vi "Thermopower-v2.vi"(0 "Gate Start":dbl format="%#_13g", 1 "hold time (sec)":dbl=10.0 format="%#_13g", 2 "Gate step - extra milliseconds to wait":u32=20000, 4 "N Gate Intervals":i32=7, 5 "Gate Step":dbl=-6.0, 6 "N Heater Intervals":i32=7, 7 "Heater Step":dbl=3.3) -> ()   [LabVIEW 2016]
uses:
  <vilib>/Utility/file.llb/Write To Spreadsheet File (DBL).vi
  <vilib>/Utility/file.llb/Read From Spreadsheet File (DBL).vi
  Driver/New driver/Agilent 415X Series.lvlib
panel:
  out "Voltage across heater (VSU 1 and SMU4) 2":dbl[][](graph)
  out "error out 2":errorcluster
  out "Gate Voltage (SMU 3) 2":dbl[](graph)
  out "Thermal Voltage (SMU2), SMU1 is Common 2":dbl[](graph)
  out "SPA VISA resource name 2":refnum<visa-resource-name>
  out "Voltage across heater (VSU 1 and SMU4)":dbl[][](graph)
  out "Gate Voltage (SMU 3)":dbl[](graph)
  out "Thermal Voltage (SMU2), SMU1 is Common":dbl[](graph)
  in  "SPA VISA resource name":refnum<visa-resource-name>="GPIB0::14::INSTR"
  in  "error in (no error)":errorcluster
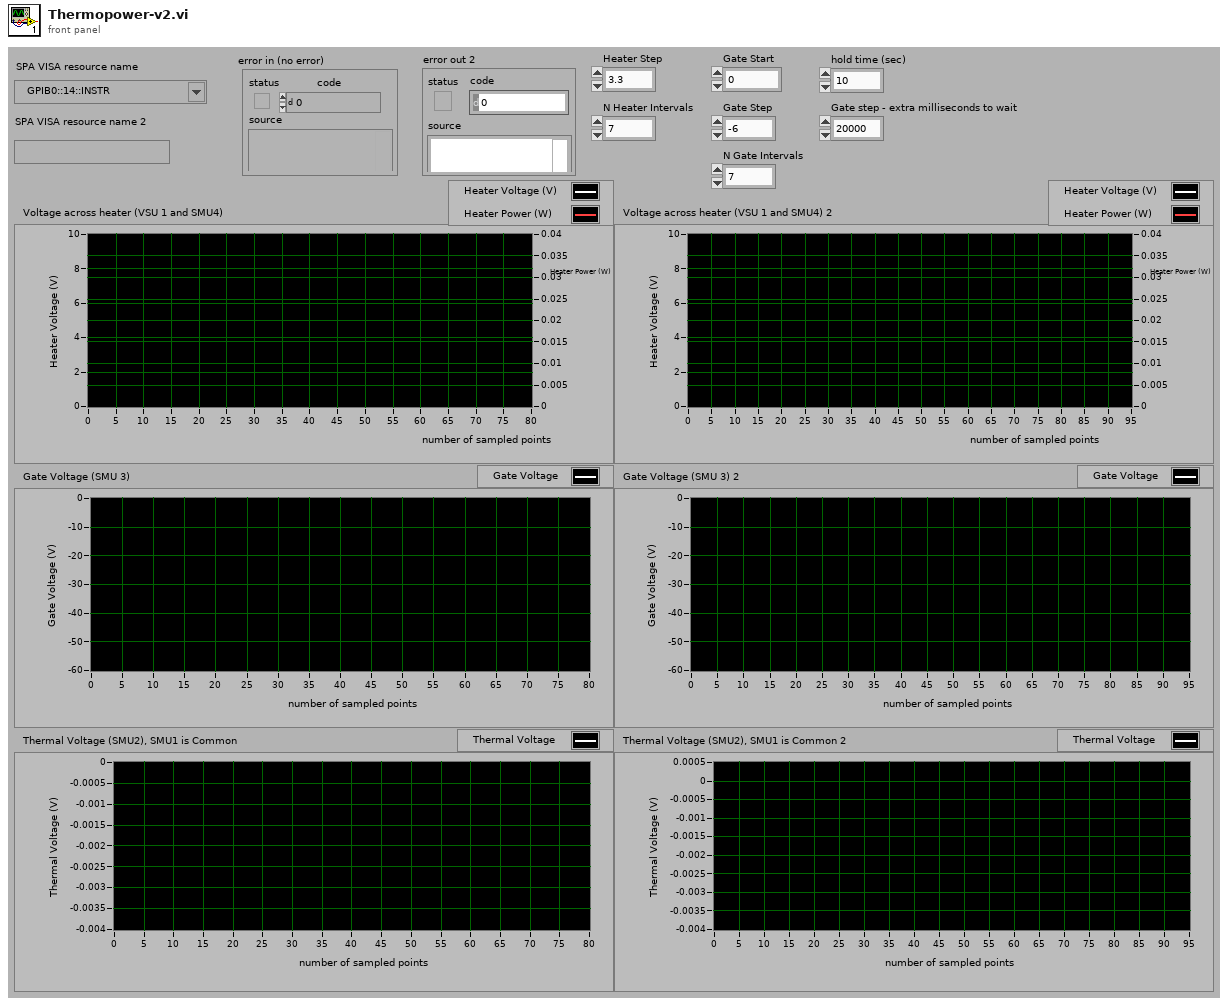
[diagram p1: front panel]
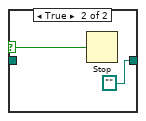
[diagram p3: hidden frame]
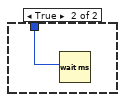
[diagram p4: hidden frame]
diagram:
  # "calculate end gate voltage"
  n1 = flat-sequence {
    tunnel: "error in (no error)" -> [w51]
    tunnel: "SPA VISA resource name" -> [w50]
    tunnel: [w49] -> w45
    tunnel: [w48] -> w44
    tunnel: w45 -> [w58]
    tunnel: w44 -> [w57]
    tunnel: [w54] -> w43
    tunnel: [w53] -> w42
    tunnel: w43 -> [w66]
    tunnel: w42 -> [w65]
    tunnel: [w64] -> w41
    tunnel: [w63] -> w40
    tunnel: w41 -> [w77]
    tunnel: w40 -> [w76]
    tunnel: [w75] -> w39
    tunnel: [w74] -> w38
    tunnel: w39 -> [w88]
    tunnel: w38 -> [w87]
    tunnel: [w86] -> w37
    tunnel: [w85] -> w35
    tunnel: w37 -> [w93]
    tunnel: [w94] -> w36
    tunnel: w35 -> [w92]
    tunnel: [w95] -> w34
    tunnel: w36 -> [w110]
    tunnel: w34 -> [w112]
    tunnel: [w111] -> w27
    tunnel: [w109] -> w26
    tunnel: w27 -> [w130]
    tunnel: w26 -> [w131]
    tunnel: [w115] -> w2
    tunnel: [w114] -> w1
    tunnel: [w133] -> w33
    tunnel: [w136] -> w32
    tunnel: [w135] -> w5
    tunnel: w2 -> [w133]
    tunnel: w1 -> [w134]
    frame #0 {
      n2 = call "Initialize.vi"("error in (no error)"=w51, "reset"=TRUE, "VISA resource name"=w50) -> ("error out"=w48:errorcluster, "VISA resource name out"=w49:refnum<visa-resource-name>)  [unwired: 2 in, 5 out]
    }
    frame #1 {
      n3 = call "Select-Meas. Mode.vi"("clear all channels"=TRUE, "error in (no error)"=w57, "measurement mode"=TRUE, "VISA resource name"=w58) -> ("error out"=w53:errorcluster, "VISA resource name out"=w54:refnum<visa-resource-name>)  [unwired: 1 in, 5 out]
    }
    frame #2 {
      w61 = 0 items=["0  ", "10K Ohms  ", "100K Ohms  ", "1M Ohms  "] ("series resistance *")
      w62 = 2 items=["V  ", "I  ", "  common  "] ("mode")
      w67 = 0 items=["SMU1  ", "SMU2  ", "SMU3  ", "SMU4  ", "SMU5  ", "SMU6  "] ("unit to configure")
      # "SMU1 configured to be common"
      n4 = call "Config-Chan-SMU-Sampling.vi"("VISA resource name in"=w66, "function"=TRUE, "series resistance *"=w61, "unit to configure"=w67, "V name (max 6 chars)"="Vgnd", "standby"=TRUE, "error in (no error)"=w65, "mode"=w62, "I name (max 6 chars)"="Ignd") -> ("VISA resource name out"=w64:refnum<visa-resource-name>, "error out"=w63:errorcluster)  [unwired: 5 out]
    }
    frame #3 {
      w71 = 0 items=["0  ", "10K Ohms  ", "100K Ohms  ", "1M Ohms  "] ("series resistance *")
      w73 = 1 items=["V  ", "I  ", "  common  "] ("mode")
      w78 = 1 items=["SMU1  ", "SMU2  ", "SMU3  ", "SMU4  ", "SMU5  ", "SMU6  "] ("unit to configure")
      # "SMU2 configured to source current (to be set to zero) \nand measure the thermal voltage"
      n5 = call "Config-Chan-SMU-Sampling.vi"("VISA resource name in"=w77, "function"=TRUE, "series resistance *"=w71, "unit to configure"=w78, "V name (max 6 chars)"="Vth", "standby"=TRUE, "error in (no error)"=w76, "mode"=w73, "I name (max 6 chars)"="Ith") -> ("VISA resource name out"=w75:refnum<visa-resource-name>, "error out"=w74:errorcluster)  [unwired: 5 out]
    }
    frame #4 {
      w82 = 0 items=["0  ", "10K Ohms  ", "100K Ohms  ", "1M Ohms  "] ("series resistance *")
      w84 = 0 items=["V  ", "I  ", "  common  "] ("mode")
      w89 = 2 items=["SMU1  ", "SMU2  ", "SMU3  ", "SMU4  ", "SMU5  ", "SMU6  "] ("unit to configure")
      # "SMU3 configured to source a gate voltage"
      n6 = call "Config-Chan-SMU-Sampling.vi"("VISA resource name in"=w88, "function"=TRUE, "series resistance *"=w82, "unit to configure"=w89, "V name (max 6 chars)"="Vg", "standby"=TRUE, "error in (no error)"=w87, "mode"=w84, "I name (max 6 chars)"="Ig") -> ("VISA resource name out"=w86:refnum<visa-resource-name>, "error out"=w85:errorcluster)  [unwired: 5 out]
    }
    frame #5 {
      w97 = 0 items=["0  ", "10K Ohms  ", "100K Ohms  ", "1M Ohms  "] ("series resistance *")
      w99 = 2 items=["V  ", "I  ", "  common  "] ("mode")
      w100 = 3 items=["SMU1  ", "SMU2  ", "SMU3  ", "SMU4  ", "SMU5  ", "SMU6  "] ("unit to configure")
      # "SMU4 configured to heater ground"
      n7 = call "Config-Chan-SMU-Sampling.vi"("VISA resource name in"=w93, "function"=TRUE, "series resistance *"=w97, "unit to configure"=w100, "V name (max 6 chars)"="Vhgnd", "standby"=TRUE, "error in (no error)"=w92, "mode"=w99, "I name (max 6 chars)"="Ihgnd") -> ("VISA resource name out"=w94:refnum<visa-resource-name>, "error out"=w95:errorcluster)  [unwired: 5 out]
    }
    frame #6 {
      # "VSU1 configured to source a voltage accross a heater"
      n8 = call "Config-Chan-VSUs-Sampling.vi"("VISA session"=w110, "VSU1 function"=TRUE, "VSU2 standby"=TRUE, "VSU1 standby"=FALSE, "VSU1 V name \n(max 6 chars)"="VSU1" ("V name (max 6 chars)"), "VSU2 V name \n(max 6 chars)"="VSU2" ("V name (max 6 chars)"), "error in (no error)"=w112, "VSU2 function"=FALSE) -> ("VISA resource name out"=w109:refnum<visa-resource-name>, "error out"=w111:errorcluster)  [unwired: 6 out]
    }
    frame #7 {
      n9 = VISA Write(VISA resource name=w131, write buffer=":PAGE:MEAS:MSET:SMU1:RANG:MODE FIX", error in (no error)=w130) -> (VISA resource name out=w129:refnum<visa-resource-name>, error out=w126:errorcluster)  [unwired: 1 out]
      n10 = VISA Write(VISA resource name=w129, write buffer=":PAGE:MEAS:MSET:SMU1:RANG 2", error in (no error)=w126) -> (VISA resource name out=w128:refnum<visa-resource-name>, error out=w125:errorcluster)  [unwired: 1 out]
      n11 = VISA Write(VISA resource name=w128, write buffer=":PAGE:MEAS:MSET:SMU2:RANG:MODE FIX", error in (no error)=w125) -> (VISA resource name out=w127:refnum<visa-resource-name>, error out=w124:errorcluster)  [unwired: 1 out]
      n12 = VISA Write(VISA resource name=w127, write buffer=":PAGE:MEAS:MSET:SMU2:RANG 2", error in (no error)=w124) -> (VISA resource name out=w119:refnum<visa-resource-name>, error out=w118:errorcluster)  [unwired: 1 out]
      n13 = VISA Write(VISA resource name=w119, write buffer=":PAGE:MEAS:MSET:ITIM LONG", error in (no error)=w118) -> (VISA resource name out=w117:refnum<visa-resource-name>, error out=w116:errorcluster)  [unwired: 1 out]
      n14 = VISA Write(VISA resource name=w117, write buffer=":PAGE:MEAS:MSET:ITIM:LONG 10", error in (no error)=w116) -> (VISA resource name out=w115:refnum<visa-resource-name>, error out=w114:errorcluster)  [unwired: 1 out]
    }
    frame #8 {
      w135 = 0.0 ("source (V or A)")
      w137 = u16 1 items=["SMU 1", "SMU2", "SMU3", "SMU4", "SMU5", "SMU6", "VSU1", "VSU2"] ("unit (SMU1:0)")
      n15 = call "Config-Sampling-Const-Source.vi"("compliance (SMUs only)"=0.0001, "error in (no error)"=w134, "source (V or A)"=w135, "unit (SMU1:0)"=w137, "VISA session"=w133) -> ("error out"=w136:errorcluster)  [unwired: 6 out]
    }
  }
  n16 = Subtract(x="N Gate Intervals", y=1) -> (x-y=w13:i32)
  n17 = Multiply(x=w13, y="Gate Step") -> (x*y=w11:dbl)
  n18 = Add(x=w11, y="Gate Start") -> (x+y=w10:dbl)
  n19 = call "File Dialog"("start path"=path "C:/users old/khk30", "pattern (all files)"="*.txt") -> ("selected path"=w30:path, "cancelled"=w29:bool)  [unwired: 10 in, 2 out]
  n20 = case shown="False" w29 {
    selector: w29 -> [_ w141]
    tunnel: w30 -> [w139 _]
    tunnel: [w139 path ""] -> w17
    frame False {
    }
    frame True {
      n21 = Stop(stop? (T)=w141) -> ()
    }
  }
  n22 = for {
    N: "N Gate Intervals" -> [_]
    tunnel: w17 -> [w153]
    tunnel: w33 -> [w152]
    tunnel: w32 -> [w151]
    tunnel: [w149] -> w21
    tunnel: [w148] -> w20
    tunnel: "N Heater Intervals" -> [w147]
    tunnel: "Gate Step" -> [w146]
    tunnel: "Gate Start" -> [w145]
    tunnel: "Heater Step" -> [w144]
    tunnel: "Gate step - extra milliseconds to wait" -> [w143]
    tunnel: [w142] -> w6 mode=indexing
    i -> [w150]
    n23 = flat-sequence {
      tunnel: w150 -> [w305]
      tunnel: [w310] -> w155
      tunnel: [w309] -> w154
      tunnel: w152 -> [w308]
      tunnel: w151 -> [w307]
      tunnel: w146 -> [w302]
      tunnel: w145 -> [w301]
      frame #0 {
        w311 = u16 2 items=["SMU 1", "SMU2", "SMU3", "SMU4", "SMU5", "SMU6", "VSU1", "VSU2"] ("unit (SMU1:0)")
        n24 = Multiply(x=w302, y=w305) -> (x*y=w304:dbl)
        n25 = Add(x=w301, y=w304) -> (x+y=w303:dbl)
        n26 = call "Config-Sampling-Const-Source.vi"("compliance (SMUs only)"=0.001, "error in (no error)"=w307, "source (V or A)"=w303, "unit (SMU1:0)"=w311, "VISA session"=w308) -> ("error out"=w309:errorcluster, "VISA resource name out"=w310:refnum<visa-resource-name>)  [unwired: 5 out]
      }
    }
    n27 = for {
      N: w147 -> [_]
      tunnel: w155 -> [w174]
      tunnel: w154 -> [w173]
      tunnel: w153 -> [w172]
      tunnel: w150 -> [w165]
      tunnel: [w160] -> w149
      tunnel: [w159] -> w148
      tunnel: w144 -> [w158]
      tunnel: w143 -> [w157]
      tunnel: [w156] -> w142 mode=indexing
      i -> [w175]
      n28 = flat-sequence {
        tunnel: [w192] -> w185
        tunnel: [w191] -> w184
        tunnel: w175 -> [w187]
        tunnel: w174 -> [w190]
        tunnel: w173 -> [w189]
        tunnel: [w187] -> w166
        tunnel: w158 -> [w186]
        tunnel: w185 -> [w202]
        tunnel: w184 -> [w200]
        tunnel: [w201] -> w183
        tunnel: [w200] -> w182
        tunnel: w166 -> [w196]
        tunnel: w165 -> [w195]
        tunnel: w157 -> [w194]
        tunnel: w183 -> [w209]
        tunnel: w182 -> [w208]
        tunnel: [w207] -> w181
        tunnel: [w206] -> w180
        tunnel: ["hold time (sec)"] -> w156
        tunnel: w181 -> [w219]
        tunnel: w180 -> [w218]
        tunnel: [w217] -> w179
        tunnel: [w216] -> w178
        tunnel: w179 -> [w225]
        tunnel: w178 -> [w224]
        tunnel: [w223] -> w177
        tunnel: [w222] -> w176
        tunnel: w177 -> [w244]
        tunnel: w176 -> [w243]
        tunnel: w172 -> [w245]
        tunnel: [w245] -> w171
        tunnel: [w245] -> w170
        tunnel: [w231] -> w168
        tunnel: [w233] -> w160
        tunnel: w171 -> [w272]
        tunnel: [w270] -> w164
        tunnel: w170 -> [w270]
        tunnel: w168 -> [w267]
        tunnel: [w267] -> w162
        tunnel: w164 -> [w276]
        tunnel: [w276] -> w163
        tunnel: w162 -> [w277]
        tunnel: [w277] -> w161
        tunnel: w163 -> [w282]
        tunnel: [w282] -> w169
        tunnel: w161 -> [w278]
        tunnel: [w278] -> w167
        tunnel: w169 -> [w296]
        tunnel: w167 -> [w287]
        tunnel: [w287] -> w159
        frame #0 {
          w193 = u16 6 items=["SMU 1", "SMU2", "SMU3", "SMU4", "SMU5", "SMU6", "VSU1", "VSU2"] ("unit (SMU1:0)")
          n29 = Multiply(x=w186, y=w187) -> (x*y=w188:dbl)
          n30 = call "Config-Sampling-Const-Source.vi"("error in (no error)"=w189, "source (V or A)"=w188, "unit (SMU1:0)"=w193, "VISA session"=w190) -> ("error out"=w192:errorcluster, "VISA resource name out"=w191:refnum<visa-resource-name>)  [unwired: 1 in, 5 out]
        }
        frame #1 {
          n31 = Equal To 0?(x=w196) -> (x = 0?=w197:bool)
          n32 = Greater Than 0?(x=w195) -> (x > 0?=w198:bool)
          n33 = And(x=w197, y=w198) -> (x .and. y?=w199:bool)
          n34 = call "Config-Display-List.vi"("error in (no error)"=w202, "list (max 8 elements)"=string[] ["Vth", "Ith", "VSU1", "Ihgnd", "Vg", "Ig", "Ignd"], "VISA session"=w200) -> ("error out"=w201:errorcluster)  [unwired: 1 in, 7 out]
          n35 = case shown="False" w199 {
            tunnel: w194 -> [_ w204]
            frame False {
            }
            frame True {
              n36 = Wait (ms)(milliseconds to wait=w204) -> ()  [unwired: 1 out]
            }
          }
        }
        frame #2 {
          w210 = 100.0  # sampling time limit
          w211 = 0 items=["linear", "log 10", "log 25", "log 50", "thinned out"] ("mode (linear: 0)")
          w212 = 0 items=["auto (linear only)", "no limit", "set limit "] ("sampling time\n(linear/thinned-out only)")
          w213 = 0.1  # initial interval (sec)
          w214 = 10  # num. of events
          w215 = 1  # number of samples
          n37 = call "Config-Sampling-Parameters.vi"("VISA session"=w208, "mode (linear: 0)"=w211, "initial interval (sec)"=w213, "sampling time\n(linear/thinned-out only)"=w212, "number of samples"=w215, "error in (no error)"=w209, "sampling time limit"=w210, "num. of events"=w214, "hold time (sec)"="hold time (sec)") -> ("VISA resource name out"=w206:refnum<visa-resource-name>, "error out"=w207:errorcluster)  [unwired: 7 in, 10 out]
        }
        frame #3 {
          w221 = 2 items=["short  ", "medium  ", "long  "] ("integration time")
          n38 = call "Config-Meas-Timing.vi"("# PLCs for long integration time"=1, "error in (no error)"=w219, "integration time"=w221, "VISA session"=w218) -> ("error out"=w217:errorcluster, "VISA resource name out"=w216:refnum<visa-resource-name>)  [unwired: 2 in, 4 out]
        }
        frame #4 {
          w227 = 1 items=["stop  ", "single  ", "single-append  ", "stress start  ", "continuous  ", "standby on  ", "standby off  ", "zero  "] ("function (stop:0)")
          n39 = call "Op-Start-Stop.vi"("time to wait (30000ms)"=600000, "error in (no error)"=w225, "function (stop:0)"=w227, "wait until finish"=TRUE, "VISA resource name"=w224) -> ("error out"=w223:errorcluster, "VISA resource name out"=w222:refnum<visa-resource-name>)  [unwired: 5 out]
        }
        frame #5 {
          # "Computes Heater power via P=VI"
          n40 = call "4155C DOWNLOAD variable.vi"("error in (no error)"=w244, "Variable name"="Vth", "VISA resource name in"=w243) -> ("error out"=w252:errorcluster, "Output data"=w239:dbl[], "VISA Resource Name out"=w257:refnum<visa-resource-name>)  [unwired: 2 out]
          n41 = call "4155C DOWNLOAD variable.vi"("error in (no error)"=w252, "Variable name"="Ith", "VISA resource name in"=w257) -> ("error out"=w251:errorcluster, "Output data"=w240:dbl[], "VISA Resource Name out"=w256:refnum<visa-resource-name>)  [unwired: 2 out]
          n42 = call "4155C DOWNLOAD variable.vi"("error in (no error)"=w251, "Variable name"="VSU1", "VISA resource name in"=w256) -> ("error out"=w250:errorcluster, "Output data"=w237:dbl[], "VISA Resource Name out"=w255:refnum<visa-resource-name>)  [unwired: 2 out]
          n43 = call "4155C DOWNLOAD variable.vi"("error in (no error)"=w250, "Variable name"="Ihgnd", "VISA resource name in"=w255) -> ("error out"=w249:errorcluster, "Output data"=w238:dbl[], "VISA Resource Name out"=w254:refnum<visa-resource-name>)  [unwired: 2 out]
          n44 = Multiply(x=w237, y=w238) -> (x*y=w242:dbl[])
          n45 = Absolute Value(x=w242) -> (abs(x)=w236:dbl[])
          n46 = call "4155C DOWNLOAD variable.vi"("error in (no error)"=w249, "Variable name"="Vg", "VISA resource name in"=w254) -> ("error out"=w248:errorcluster, "Output data"=w241:dbl[], "VISA Resource Name out"=w253:refnum<visa-resource-name>)  [unwired: 2 out]
          n47 = call "4155C DOWNLOAD variable.vi"("error in (no error)"=w248, "Variable name"="Ig", "VISA resource name in"=w253) -> ("error out"=w232:errorcluster, "Output data"=w230:dbl[], "VISA Resource Name out"=w235:refnum<visa-resource-name>)  [unwired: 2 out]
          n48 = call "4155C DOWNLOAD variable.vi"("error in (no error)"=w232, "Variable name"="Ignd", "VISA resource name in"=w235) -> ("error out"=w231:errorcluster, "Output data"=w229:dbl[], "VISA Resource Name out"=w233:refnum<visa-resource-name>)  [unwired: 2 out]
          n49 = Build Array(w236, w237, w238, w239, w240, w241, w230, w229) -> (w247:dbl[][])
          n50 = call-poly <vilib>:"Write To Spreadsheet File.vi"("transpose? (no:F)"=TRUE, "format (%.3f)"="%.13f", "append to file? (new file:F)"=TRUE, "2D data"=w247, "file path (dialog if empty)"=w245) -> ()  [unwired: 1 in, 3 out]
        }
        frame #6 {
          # "plot the thermal voltage after reading the file"
          n51 = call-poly <vilib>:"Read From Spreadsheet File.vi"("transpose (no:F)"=TRUE, "format (%.3f)"="%.13f", "max characters/row  (no limit:0)"=0, "number of rows (all:-1)"=-1, "file path (dialog if empty)"=w272) -> ("all rows"=w269:dbl[][])  [unwired: 6 out]
          n52 = Index Array(array=w269, index (row)=3) -> (element=→"Thermal Voltage (SMU2), SMU1 is Common":dbl[])  [unwired: 1 in]
        }
        frame #7 {
        }
        frame #8 {
          # "plot the gate voltage after reading the file"
          n53 = call-poly <vilib>:"Read From Spreadsheet File.vi"("transpose (no:F)"=TRUE, "format (%.3f)"="%.13f", "max characters/row  (no limit:0)"=0, "number of rows (all:-1)"=-1, "file path (dialog if empty)"=w282) -> ("all rows"=w281:dbl[][])  [unwired: 6 out]
          n54 = Index Array(array=w281, index (row)=5) -> (element=→"Gate Voltage (SMU 3)":dbl[])  [unwired: 1 in]
        }
        frame #9 {
          # "plot the voltage across the heater and the \npower dissipated by the heater after reading the file"
          n55 = call-poly <vilib>:"Read From Spreadsheet File.vi"("transpose (no:F)"=TRUE, "format (%.3f)"="%.13f", "max characters/row  (no limit:0)"=0, "number of rows (all:-1)"=-1, "file path (dialog if empty)"=w296) -> ("all rows"=w294:dbl[][])  [unwired: 6 out]
          n56 = Index Array(array=w294, index (row)=1) -> (element=w288:dbl[])  [unwired: 1 in]
          n57 = Index Array(array=w294, index (row)=2) -> (element=w292:dbl[])  [unwired: 1 in]
          n58 = Multiply(x=w288, y=w292) -> (x*y=w291:dbl[])
          n59 = Absolute Value(x=w291) -> (abs(x)=w290:dbl[])
          n60 = Build Array(w288, w290) -> (→"Voltage across heater (VSU 1 and SMU4)":dbl[][])
        }
      }
    }
  }
  n61 = flat-sequence {
    tunnel: [w319] -> w25
    tunnel: [w318] -> w24
    tunnel: w21 -> [w313]
    tunnel: w20 -> [w312]
    tunnel: w25 -> [w330]
    tunnel: w24 -> [w329]
    tunnel: [w324] -> w4
    tunnel: [w323] -> w3
    tunnel: [w334] -> w23
    tunnel: [w335] -> w22
    tunnel: w4 -> [w337]
    tunnel: w3 -> [w336]
    tunnel: w23 -> [w351]
    tunnel: w22 -> [w352]
    tunnel: [w350] -> w18
    tunnel: [w349] -> w19
    tunnel: w5 -> [w348]
    frame #0 {
      w316 = 0 items=["0  ", "10K Ohms  ", "100K Ohms  ", "1M Ohms  "] ("series resistance *")
      w317 = 2 items=["V  ", "I  ", "  common  "] ("mode")
      w320 = 1 items=["SMU1  ", "SMU2  ", "SMU3  ", "SMU4  ", "SMU5  ", "SMU6  "] ("unit to configure")
      # "SMU2 configured to be common"
      n62 = call "Config-Chan-SMU-Sampling.vi"("VISA resource name in"=w313, "function"=TRUE, "series resistance *"=w316, "unit to configure"=w320, "V name (max 6 chars)"="Vgnd", "standby"=TRUE, "error in (no error)"=w312, "mode"=w317, "I name (max 6 chars)"="Ignd") -> ("VISA resource name out"=w319:refnum<visa-resource-name>, "error out"=w318:errorcluster)  [unwired: 5 out]
    }
    frame #1 {
      w326 = 0 items=["0  ", "10K Ohms  ", "100K Ohms  ", "1M Ohms  "] ("series resistance *")
      w328 = 1 items=["V  ", "I  ", "  common  "] ("mode")
      w331 = 0 items=["SMU1  ", "SMU2  ", "SMU3  ", "SMU4  ", "SMU5  ", "SMU6  "] ("unit to configure")
      # "SMU2 configured to source current (to be set to zero) \nand measure the thermal voltage"
      n63 = call "Config-Chan-SMU-Sampling.vi"("VISA resource name in"=w330, "function"=TRUE, "series resistance *"=w326, "unit to configure"=w331, "V name (max 6 chars)"="Vth", "standby"=TRUE, "error in (no error)"=w329, "mode"=w328, "I name (max 6 chars)"="Ith") -> ("VISA resource name out"=w324:refnum<visa-resource-name>, "error out"=w323:errorcluster)  [unwired: 5 out]
    }
    frame #2 {
      n64 = VISA Write(VISA resource name=w337, write buffer=":PAGE:MEAS:MSET:SMU1:RANG:MODE FIX", error in (no error)=w336) -> (VISA resource name out=w346:refnum<visa-resource-name>, error out=w343:errorcluster)  [unwired: 1 out]
      n65 = VISA Write(VISA resource name=w346, write buffer=":PAGE:MEAS:MSET:SMU1:RANG 2", error in (no error)=w343) -> (VISA resource name out=w345:refnum<visa-resource-name>, error out=w342:errorcluster)  [unwired: 1 out]
      n66 = VISA Write(VISA resource name=w345, write buffer=":PAGE:MEAS:MSET:SMU2:RANG:MODE FIX", error in (no error)=w342) -> (VISA resource name out=w344:refnum<visa-resource-name>, error out=w341:errorcluster)  [unwired: 1 out]
      n67 = VISA Write(VISA resource name=w344, write buffer=":PAGE:MEAS:MSET:SMU2:RANG 2", error in (no error)=w341) -> (VISA resource name out=w335:refnum<visa-resource-name>, error out=w334:errorcluster)  [unwired: 1 out]
    }
    frame #3 {
      w353 = u16 0 items=["SMU 1", "SMU2", "SMU3", "SMU4", "SMU5", "SMU6", "VSU1", "VSU2"] ("unit (SMU1:0)")
      n68 = call "Config-Sampling-Const-Source.vi"("compliance (SMUs only)"=0.0001, "error in (no error)"=w351, "source (V or A)"=w348, "unit (SMU1:0)"=w353, "VISA session"=w352) -> ("error out"=w349:errorcluster, "VISA resource name out"=w350:refnum<visa-resource-name>)  [unwired: 5 out]
    }
  }
  n69 = for {
    N: "N Gate Intervals" -> [_]
    tunnel: w17 -> [w366]
    tunnel: w18 -> [w365]
    tunnel: w19 -> [w364]
    tunnel: [w362] -> _
    tunnel: [w361] -> _
    tunnel: "N Heater Intervals" -> [w360]
    tunnel: w10 -> [w359]
    tunnel: "Gate Step" -> [w358]
    tunnel: "Heater Step" -> [w357]
    tunnel: "Gate step - extra milliseconds to wait" -> [w356]
    tunnel: w6 -> [w355] mode=indexing
    i -> [w363]
    n70 = flat-sequence {
      tunnel: w363 -> [w523]
      tunnel: [w528] -> w368
      tunnel: [w527] -> w367
      tunnel: w365 -> [w526]
      tunnel: w364 -> [w525]
      tunnel: w359 -> [w521]
      tunnel: w358 -> [w519]
      frame #0 {
        w529 = u16 2 items=["SMU 1", "SMU2", "SMU3", "SMU4", "SMU5", "SMU6", "VSU1", "VSU2"] ("unit (SMU1:0)")
        n71 = Multiply(x=w519, y=w523) -> (x*y=w520:dbl)
        n72 = Subtract(x=w521, y=w520) -> (x-y=w522:dbl)
        n73 = call "Config-Sampling-Const-Source.vi"("compliance (SMUs only)"=0.001, "error in (no error)"=w525, "source (V or A)"=w522, "unit (SMU1:0)"=w529, "VISA session"=w526) -> ("error out"=w527:errorcluster, "VISA resource name out"=w528:refnum<visa-resource-name>)  [unwired: 5 out]
      }
    }
    n74 = for {
      N: w360 -> [_]
      tunnel: w368 -> [w387]
      tunnel: w367 -> [w386]
      tunnel: w366 -> [w385]
      tunnel: w363 -> [w378]
      tunnel: [w373] -> w362
      tunnel: [w372] -> w361
      tunnel: w357 -> [w371]
      tunnel: w356 -> [w370]
      tunnel: w355 -> [w369] mode=indexing
      i -> [w388]
      n75 = flat-sequence {
        tunnel: [w405] -> w398
        tunnel: [w404] -> w397
        tunnel: w388 -> [w400]
        tunnel: w387 -> [w403]
        tunnel: w386 -> [w402]
        tunnel: [w400] -> w379
        tunnel: w371 -> [w399]
        tunnel: w398 -> [w415]
        tunnel: w397 -> [w413]
        tunnel: [w414] -> w396
        tunnel: [w413] -> w395
        tunnel: w379 -> [w409]
        tunnel: w378 -> [w408]
        tunnel: w370 -> [w407]
        tunnel: w396 -> [w422]
        tunnel: w395 -> [w421]
        tunnel: [w420] -> w394
        tunnel: [w419] -> w393
        tunnel: w369 -> [w418]
        tunnel: w394 -> [w432]
        tunnel: w393 -> [w431]
        tunnel: [w430] -> w392
        tunnel: [w429] -> w391
        tunnel: w392 -> [w438]
        tunnel: w391 -> [w437]
        tunnel: [w436] -> w390
        tunnel: [w435] -> w389
        tunnel: w390 -> [w457]
        tunnel: w389 -> [w456]
        tunnel: w385 -> [w458]
        tunnel: [w458] -> w384
        tunnel: [w458] -> w383
        tunnel: [w445] -> w381
        tunnel: [w444] -> w373
        tunnel: w384 -> [w485]
        tunnel: [w483] -> w377
        tunnel: w383 -> [w483]
        tunnel: w381 -> [w480]
        tunnel: [w480] -> w375
        tunnel: w377 -> [w489]
        tunnel: [w489] -> w376
        tunnel: w375 -> [w490]
        tunnel: [w490] -> w374
        tunnel: w376 -> [w495]
        tunnel: [w495] -> w382
        tunnel: w374 -> [w491]
        tunnel: [w491] -> w380
        tunnel: w382 -> [w514]
        tunnel: w380 -> [w500]
        tunnel: [w500] -> w372
        frame #0 {
          w406 = u16 6 items=["SMU 1", "SMU2", "SMU3", "SMU4", "SMU5", "SMU6", "VSU1", "VSU2"] ("unit (SMU1:0)")
          n76 = Multiply(x=w399, y=w400) -> (x*y=w401:dbl)
          n77 = call "Config-Sampling-Const-Source.vi"("error in (no error)"=w402, "source (V or A)"=w401, "unit (SMU1:0)"=w406, "VISA session"=w403) -> ("error out"=w405:errorcluster, "VISA resource name out"=w404:refnum<visa-resource-name>)  [unwired: 1 in, 5 out]
        }
        frame #1 {
          n78 = Equal To 0?(x=w409) -> (x = 0?=w410:bool)
          n79 = Greater Than 0?(x=w408) -> (x > 0?=w411:bool)
          n80 = And(x=w410, y=w411) -> (x .and. y?=w412:bool)
          n81 = call "Config-Display-List.vi"("error in (no error)"=w415, "list (max 8 elements)"=string[] ["Vth", "Ith", "VSU1", "Ihgnd", "Vg", "Ig", "Ignd"], "VISA session"=w413) -> ("error out"=w414:errorcluster)  [unwired: 1 in, 7 out]
          n82 = case shown="True" w412 {
            tunnel: w407 -> [_ w417]
            frame False {
            }
            frame True {
              n83 = Wait (ms)(milliseconds to wait=w417) -> ()  [unwired: 1 out]
            }
          }
        }
        frame #2 {
          w423 = 100.0  # sampling time limit
          w424 = 0 items=["linear", "log 10", "log 25", "log 50", "thinned out"] ("mode (linear: 0)")
          w425 = 0 items=["auto (linear only)", "no limit", "set limit "] ("sampling time\n(linear/thinned-out only)")
          w426 = 0.1  # initial interval (sec)
          w427 = 10  # num. of events
          w428 = 1  # number of samples
          n84 = call "Config-Sampling-Parameters.vi"("VISA session"=w421, "mode (linear: 0)"=w424, "initial interval (sec)"=w426, "sampling time\n(linear/thinned-out only)"=w425, "number of samples"=w428, "error in (no error)"=w422, "sampling time limit"=w423, "num. of events"=w427, "hold time (sec)"=w418) -> ("VISA resource name out"=w419:refnum<visa-resource-name>, "error out"=w420:errorcluster)  [unwired: 7 in, 10 out]
        }
        frame #3 {
          w434 = 2 items=["short  ", "medium  ", "long  "] ("integration time")
          n85 = call "Config-Meas-Timing.vi"("# PLCs for long integration time"=1, "error in (no error)"=w432, "integration time"=w434, "VISA session"=w431) -> ("error out"=w430:errorcluster, "VISA resource name out"=w429:refnum<visa-resource-name>)  [unwired: 2 in, 4 out]
        }
        frame #4 {
          w440 = 1 items=["stop  ", "single  ", "single-append  ", "stress start  ", "continuous  ", "standby on  ", "standby off  ", "zero  "] ("function (stop:0)")
          n86 = call "Op-Start-Stop.vi"("time to wait (30000ms)"=600000, "error in (no error)"=w438, "function (stop:0)"=w440, "wait until finish"=TRUE, "VISA resource name"=w437) -> ("error out"=w436:errorcluster, "VISA resource name out"=w435:refnum<visa-resource-name>)  [unwired: 5 out]
        }
        frame #5 {
          # "Computes Heater power via P=VI"
          n87 = call "4155C DOWNLOAD variable.vi"("error in (no error)"=w457, "Variable name"="Vth", "VISA resource name in"=w456) -> ("error out"=w465:errorcluster, "Output data"=w451:dbl[], "VISA Resource Name out"=w470:refnum<visa-resource-name>)  [unwired: 2 out]
          n88 = call "4155C DOWNLOAD variable.vi"("error in (no error)"=w465, "Variable name"="Ith", "VISA resource name in"=w470) -> ("error out"=w464:errorcluster, "Output data"=w452:dbl[], "VISA Resource Name out"=w469:refnum<visa-resource-name>)  [unwired: 2 out]
          n89 = call "4155C DOWNLOAD variable.vi"("error in (no error)"=w464, "Variable name"="VSU1", "VISA resource name in"=w469) -> ("error out"=w463:errorcluster, "Output data"=w449:dbl[], "VISA Resource Name out"=w468:refnum<visa-resource-name>)  [unwired: 2 out]
          n90 = call "4155C DOWNLOAD variable.vi"("error in (no error)"=w463, "Variable name"="Ihgnd", "VISA resource name in"=w468) -> ("error out"=w462:errorcluster, "Output data"=w450:dbl[], "VISA Resource Name out"=w467:refnum<visa-resource-name>)  [unwired: 2 out]
          n91 = Multiply(x=w449, y=w450) -> (x*y=w455:dbl[])
          n92 = Absolute Value(x=w455) -> (abs(x)=w448:dbl[])
          n93 = call "4155C DOWNLOAD variable.vi"("error in (no error)"=w462, "Variable name"="Vg", "VISA resource name in"=w467) -> ("error out"=w461:errorcluster, "Output data"=w453:dbl[], "VISA Resource Name out"=w466:refnum<visa-resource-name>)  [unwired: 2 out]
          n94 = call "4155C DOWNLOAD variable.vi"("error in (no error)"=w461, "Variable name"="Ig", "VISA resource name in"=w466) -> ("error out"=w446:errorcluster, "Output data"=w454:dbl[], "VISA Resource Name out"=w447:refnum<visa-resource-name>)  [unwired: 2 out]
          n95 = call "4155C DOWNLOAD variable.vi"("error in (no error)"=w446, "Variable name"="Ignd", "VISA resource name in"=w447) -> ("error out"=w445:errorcluster, "Output data"=w443:dbl[], "VISA Resource Name out"=w444:refnum<visa-resource-name>)  [unwired: 2 out]
          "SPA VISA resource name 2" <- w444
          n96 = Build Array(w448, w449, w450, w451, w452, w453, w454, w443) -> (w460:dbl[][])
          n97 = call-poly <vilib>:"Write To Spreadsheet File.vi"("transpose? (no:F)"=TRUE, "format (%.3f)"="%.13f", "append to file? (new file:F)"=TRUE, "2D data"=w460, "file path (dialog if empty)"=w458) -> ()  [unwired: 1 in, 3 out]
        }
        frame #6 {
          # "plot the thermal voltage after reading the file"
          n98 = call-poly <vilib>:"Read From Spreadsheet File.vi"("transpose (no:F)"=TRUE, "format (%.3f)"="%.13f", "max characters/row  (no limit:0)"=0, "number of rows (all:-1)"=-1, "file path (dialog if empty)"=w485) -> ("all rows"=w482:dbl[][])  [unwired: 6 out]
          n99 = Index Array(array=w482, index (row)=3) -> (element=→"Thermal Voltage (SMU2), SMU1 is Common 2":dbl[])  [unwired: 1 in]
        }
        frame #7 {
        }
        frame #8 {
          # "plot the gate voltage after reading the file"
          n100 = call-poly <vilib>:"Read From Spreadsheet File.vi"("transpose (no:F)"=TRUE, "format (%.3f)"="%.13f", "max characters/row  (no limit:0)"=0, "number of rows (all:-1)"=-1, "file path (dialog if empty)"=w495) -> ("all rows"=w494:dbl[][])  [unwired: 6 out]
          n101 = Index Array(array=w494, index (row)=5) -> (element=→"Gate Voltage (SMU 3) 2":dbl[])  [unwired: 1 in]
        }
        frame #9 {
          # "plot the voltage across the heater and the \npower dissipated by the heater after reading the file"
          n102 = call-poly <vilib>:"Read From Spreadsheet File.vi"("transpose (no:F)"=TRUE, "format (%.3f)"="%.13f", "max characters/row  (no limit:0)"=0, "number of rows (all:-1)"=-1, "file path (dialog if empty)"=w514) -> ("all rows"=w512:dbl[][])  [unwired: 6 out]
          n103 = Index Array(array=w512, index (row)=1) -> (element=w506:dbl[])  [unwired: 1 in]
          n104 = Index Array(array=w512, index (row)=2) -> (element=w510:dbl[])  [unwired: 1 in]
          n105 = property on="Voltage across heater (VSU 1 and SMU4) 2" class="WFGraph (strict)"(error in=w500, "Active Plot"=u32 0, "Plot.YScaleIdx"=u32 0 ("Plot.Y Scale Index"), "Active Plot"=u32 1, "Plot.YScaleIdx"=u32 1 ("Plot.Y Scale Index")) -> (error out=→"error out 2":errorcluster)  [unwired: 1 in, 1 out]
          n106 = Multiply(x=w506, y=w510) -> (x*y=w509:dbl[])
          n107 = Absolute Value(x=w509) -> (abs(x)=w508:dbl[])
          n108 = Build Array(w506, w508) -> (→"Voltage across heater (VSU 1 and SMU4) 2":dbl[][])
        }
      }
    }
  }
